vi "Rotate Array 2012 NIVerified.vi"(6 "Rotation CW/nCCW":bool, 9 "Rotation":enum8{"90", "180", "270", "0"}(ring), 11 "Array":dbl[][](array[numeric])=[[0.0, 1.0, 2.0, 12.0], [3.0, 4.0, 5.0, 12.0], [6.0, 7.0, 8.0, 12.0], [9.0, 10.0, 11.0, 12.0]]) -> (1 "Rotated 2D Array":dbl[][](array[numeric]))   [LabVIEW 2020]
doc: "This VI rotates a 2D array in either clockwise or clockwise by a multiple of 90 degrees."
panel:
  # "Overview: This VI rotates a 2D array either clockwise or counterclockwise by 90, 180, or 270 degrees.\nRequirements: LabVIEW Base Development System\nInstructions:\n1. Select Rotation orientation.\n2. Run the VI.\n3. Inspect Rotated 2D Array indicator."
  # "Clockwise"
  # "Counterclockwise"
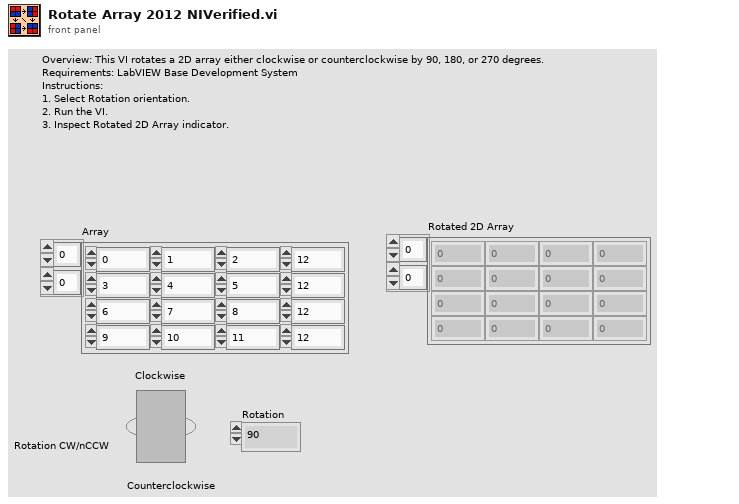
[diagram p1: front panel]
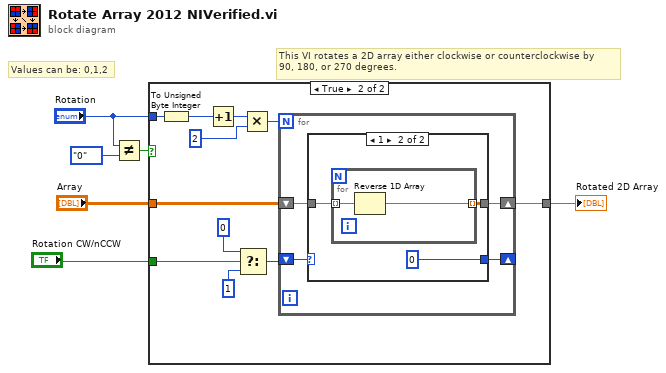
[diagram p0: block diagram]
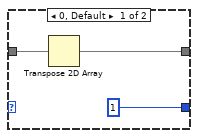
[diagram p3: hidden frame]
diagram:
  # "Values can be: 0,1,2"
  # "This VI rotates a 2D array either clockwise or counterclockwise by\n90, 180, or 270 degrees."
  n1 = Not Equal?(x="Rotation", y=enum8{"90", "180", "270", "0"}."0") -> (x != y?=w3:bool)
  n2 = case shown="True" w3 {
    tunnel: "Array" -> [w7 w18]
    tunnel: [w7 w17] -> w5
    tunnel: "Rotation" -> [_ w16]
    tunnel: "Rotation CW/nCCW" -> [_ w15]
    frame False {
    }
    frame True {
      n3 = To Unsigned Byte Integer(number=w16) -> (unsigned 8bit integer=w8:u8)
      n4 = Increment(x=w8) -> (x+1=w10:u8)
      n5 = Select(t=u8 0, s=w15, f=u8 1) -> (s? t:f=w12:u8)
      n6 = Multiply(x=w10, y=u8 2) -> (x*y=w11:u8)
      n7 = for {
        N: w11 -> [_]
        shift-right: [w21] -> w17
        shift-left: w18 -> [w22]
        shift-right: [w19] -> _
        shift-left: w12 -> [w20]
        n8 = case shown="1" w20 {
          tunnel: w22 -> [w24 w28]
          tunnel: [w25 w27] -> w21
          tunnel: [u8 1 u8 0] -> w19
          frame 0, Default {
            n9 = Transpose 2D Array(2D array=w24) -> (transposed array=w25:dbl[][])
          }
          frame 1 {
            n10 = for {
              tunnel: w28 -> [w30] mode=indexing
              tunnel: [w29] -> w27 mode=indexing
              n11 = Reverse 1D Array(array=w30) -> (reversed array=w29:dbl[])
            }
          }
        }
      }
    }
  }
  "Rotated 2D Array" <- w5
